vi "GetNI_SynthFocus_Bulk.vi"(0 "Digitizer Settings":T4={"Digitizer delay (us) "=0.0, "rf points per line"=2048, "lines per plane"=128, "Samp Rate (Hz)"=100000000.0, "Additional dig delay (us)"=0.0, "Voltage Scale"=0.4, "Pre-Looks"=0, "Offset delay (us)"=0.0, "bits A/D"=8, "Avg Num"=1, "DigTimeOut"=5.0, "Rel Dig Delay"=0.0, "Dig Ch"=0, "LeCroyCluster"={"LeCroy Channels"=[TRUE, FALSE, FALSE, FALSE], "LC read pt offset"=0.0, "Sweep Avg"=FALSE}, "Main Digitizer"=enum."NI Digitizer", "Dig Config"=enum."Single channel", "Digitizer ID Cluster"={"Acqiris/Alazar/SP ID"=[], "NI Instr Handles"=[], "LeCroy VISA"="", "GaGe Handle"={"Handle"=0, "Sample size"=0, "Resolution"=0, "Offset"=0, "Channels"=0, "Boards"=0}, "ATS Ref"="ATS9350", "Acqiris Address"=["PCI::INSTR0"], "ADQRef"=refnum, "adq_cu_ptr"=refnum}, "Trigger Settings"={"Trig Source"=1, "Trig Coupling"=0, "Trig Slope"=0, "Level (mV)"=1500.0}, "Bulk Acq"=FALSE, "Bulk Start Indexes"=[], "Data Ref RF"=refnum, "NI ID/Channel"=[], "Total Dig CH"=1, "Xtra Ann Trig delay (us)"=10.0, "Fix Z Delay?"=FALSE, "One Way Transmission?"=FALSE, "Data Ref Log"=refnum} {"Trigger Settings"."Trig Slope" items=["Positive", "Negative"]; "Trigger Settings"."Level (mV)" format="%.2f"; "Trigger Settings"."Trig Coupling" items=["DC 1 MOhm", "AC 1 MOhm", "DC 50 Ohm", "AC 50 Ohm"]; "Trigger Settings"."Trig Source" items=["Chan 1", "External"]; "Rel Dig Delay" format="%.2f"; "DigTimeOut" format="%.2f"; "Avg Num" min=1; "Offset delay (us)" format="%.2f"; "Additional dig delay (us)" format="%.2f"; "Digitizer delay (us)" format="%.2f"}, 5 "Ann Array Params":T1={"Synth Foc?"=FALSE, "Focal Zones"=41, "Switch T/R"=0, "Trans Geometry (mm)"={"Transducer"=0, "Geo Focus"=12.0, "a (radius)"=3.0, "# of rings"=5, "kerf space "=0.1, "Center Freq"=12.0}, "Sub Ap Excite?"=FALSE, "Full Array Scan?"=FALSE, "Xmt/Rcv"={"XMIT"=[TRUE, TRUE, TRUE, TRUE, TRUE], "RCV"=[TRUE, TRUE, TRUE, TRUE, TRUE]}, "PulseSpacing (us)"=0.0, "Xmit Ring"=0, "XMIT CHS"=0, "RCV CHS"=0, "GPU?"=FALSE, "Save TIFF?"=FALSE, "downfactor"=1, "RCV 1CH"=0} {"RCV 1CH" items=["All", "1", "2", "3", "4", "5"]; "Trans Geometry (mm)"."Transducer" items=["6D 12R 40 MHz"=0, "10D 31R 20 MHz"=1, "10D 23R 20 MHz"=2, "6D 23R 40 MHz"=3, "4.5D 10.7R 40 MHz"=4, "9D 23.5R 20 MHz"=5, "9D 25.8R 20MHz"=6, "Enter"=99]; "Switch T/R" min=1 max=5 step=1}, 7 "errorin":errorcluster, 8 "File Array":string[](array[string]), 10 "lines per plane":i32) -> (17 "Raw VGain (scale)":dbl, 18 "Gain Array":T8(array[cluster]), 21 "VGain (dB)":dbl, 27 "error out":errorcluster)   [LabVIEW 2022 SP3]
uses:
  -DigitizerRoutines/DigitizerSettings.ctl
  -DigitizerRoutines/Digitizer.ctl
  -DigitizerRoutines/DigConfig.ctl
  -DigitizerRoutines/DigitizerID.ctl
  C:/Windows/System32/ADQAPI_dotNet_helper.dll
  Annular Array/-AnnularRoutines/AnnularArray.ctl
  Annular Array/-AnnularRoutines/TransGeometry.ctl
  Annular Array/-AnnularRoutines/ArrayGeometry.ctl
  <instrlib>/niScope/Acquire/Fetch/niScope Multi Fetch Binary 8.vi
  -ScanSystem/DataHandling/ReverseDataI8.vi
  Annular Array/-SynthApperture/ProcImageHD_I8.vi
panel:
  out "read time":u32
  out "synth foc time":u32
  out "Numeric":i32
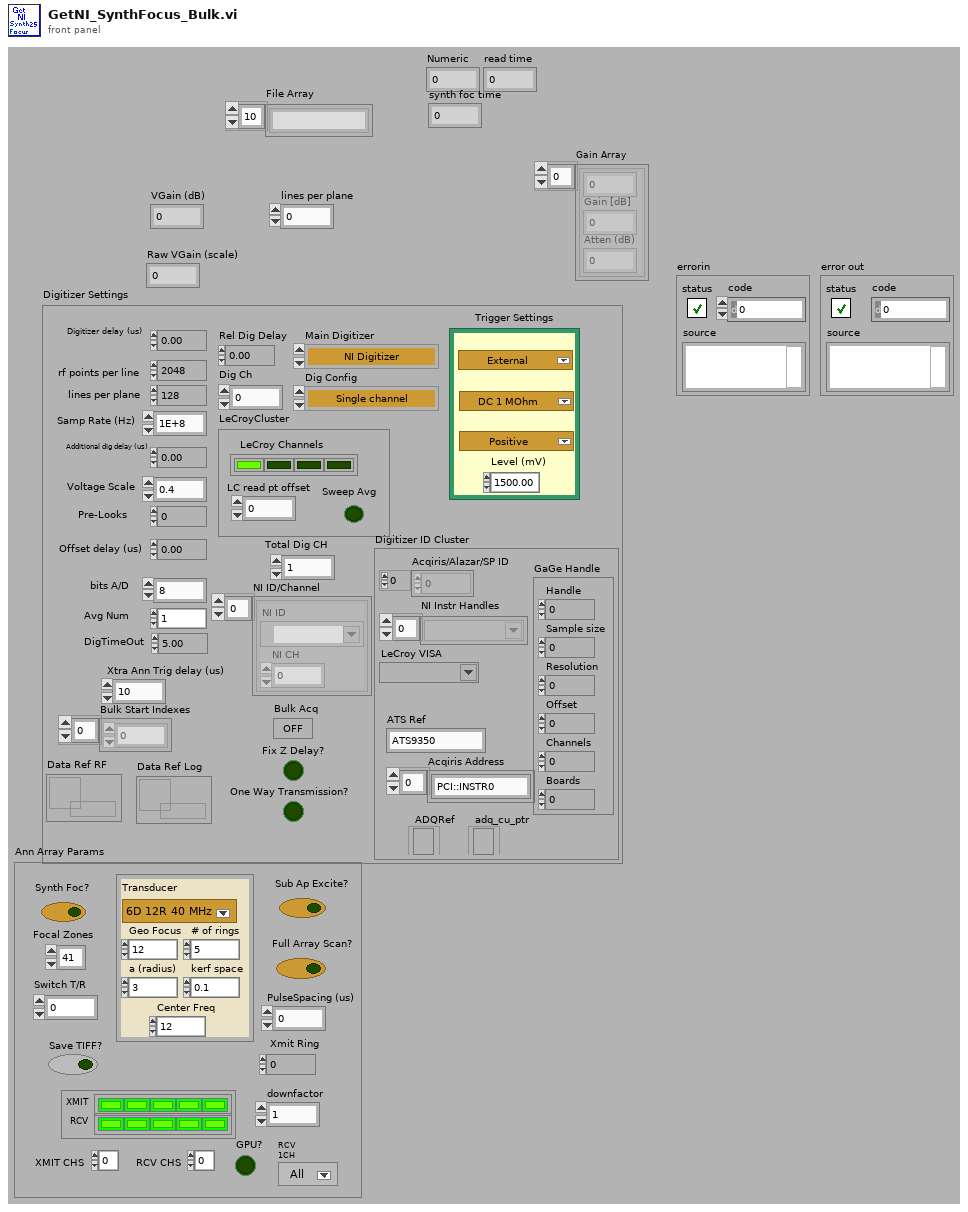
[diagram p1: front panel]
types:
  T1 = typedef "AnnularArray.ctl" = cluster{"Synth Foc?":bool, "Focal Zones":i16, "Switch T/R":i16, "Trans Geometry (mm)":T2, "Sub Ap Excite?":bool, "Full Array Scan?":bool, "Xmt/Rcv":cluster{"XMIT":bool[], "RCV":bool[]}, "PulseSpacing (us)":sgl, "Xmit Ring":i32, "XMIT CHS":u8, "RCV CHS":u8, "GPU?":bool, "Save TIFF?":bool, "downfactor":i32, "RCV 1CH":u16}
  T2 = typedef "TransGeometry.ctl" = cluster{"Transducer":T3, "Geo Focus":dbl, "a (radius)":dbl, "# of rings":i32, "kerf space ":dbl, "Center Freq":dbl}
  T3 = typedef "ArrayGeometry.ctl" = u16
  T4 = typedef "DigitizerSettings.ctl" = cluster{"Digitizer delay (us) ":dbl, "rf points per line":i32, "lines per plane":i32, "Samp Rate (Hz)":dbl, "Additional dig delay (us)":dbl, "Voltage Scale":dbl, "Pre-Looks":i32, "Offset delay (us)":dbl, "bits A/D":i8, "Avg Num":i32, "DigTimeOut":sgl, "Rel Dig Delay":sgl, "Dig Ch":i32, "LeCroyCluster":cluster{"LeCroy Channels":bool[], "LC read pt offset":dbl, "Sweep Avg":bool}, "Main Digitizer":T5, "Dig Config":T6, "Digitizer ID Cluster":T7, "Trigger Settings":cluster{"Trig Source":u16, "Trig Coupling":u16, "Trig Slope":u16, "Level (mV)":dbl}, "Bulk Acq":bool, "Bulk Start Indexes":i32[], "Data Ref RF":refnum<data-value>, "NI ID/Channel":cluster{"NI ID":refnum<k15>, "NI CH":i32}[], "Total Dig CH":i32, "Xtra Ann Trig delay (us)":dbl, "Fix Z Delay?":bool, "One Way Transmission?":bool, "Data Ref Log":refnum<data-value>}
  T5 = typedef "Digitizer.ctl" = enum16{"Acqiris Digitizer", "NI Digitizer", "LeCroy", "GaGe", "AlazarTech", "No Digitizer", "Teledyne"}
  T6 = typedef "DigConfig.ctl" = enum16{"Single channel", "2 Chans w/ 2 Acqiris", "2 Chans w/ 1 Acqiris", "5-CH Pulser New", "5-CH pulser w/ ann array", "5-pass style ann array", "Empty"}
  T7 = typedef "DigitizerID.ctl" = cluster{"Acqiris/Alazar/SP ID":u32[], "NI Instr Handles":refnum<k15>[], "LeCroy VISA":refnum<visa-resource-name>, "GaGe Handle":cluster{"Handle":u32, "Sample size":u32, "Resolution":i32, "Offset":i32, "Channels":u32, "Boards":u32}, "ATS Ref":string, "Acqiris Address":string[], "ADQRef":refnum<k24>, "adq_cu_ptr":refnum<k24>}
  T8 = cluster{sgl, "Gain [dB]  ":sgl, "Atten (dB)":sgl}[]
  T9 = cluster{"gain":dbl, "wfm":i8[][], "max queue size (-1, unlimited)":i32}
  T10 = cluster{"actualSamples":i32, "absoluteInitialX":dbl, "relativeInitialX":dbl, "xIncrement":dbl, "offset":dbl, "gain":dbl, "reserved1":dbl, "reserved2":dbl}[]
  T11 = cluster{"actualSamples":i32, "absoluteInitialX":dbl, "relativeInitialX":dbl, "xIncrement":dbl, "offset":dbl, "gain":dbl, "reserved1":dbl, "reserved2":dbl}
  T12 = cluster{sgl, "Gain [dB]  ":sgl, "Atten (dB)":sgl}
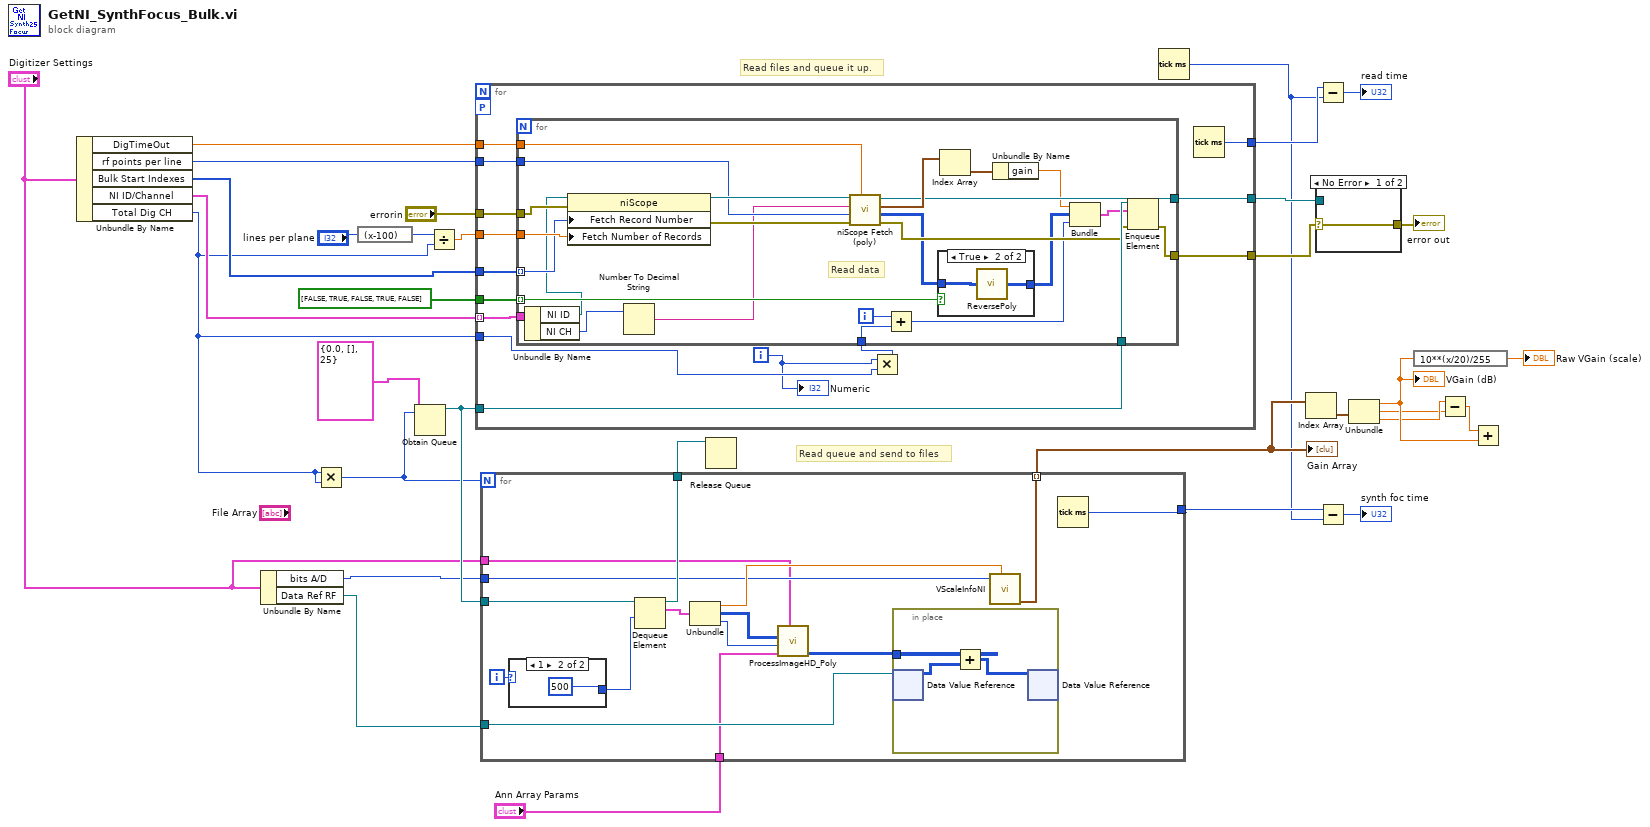
[diagram p0: block diagram]
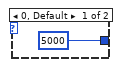
[diagram p2: hidden frame]
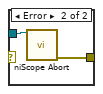
[diagram p3: hidden frame]
diagram:
  # "Read files and queue it up."
  # "Read queue and send to files"
  n1 = Unbundle By Name("Digitizer Settings") -> ("DigTimeOut"=w10:sgl, "rf points per line"=w12:i32, "Bulk Start Indexes"=w8:i32[], "NI ID/Channel"=w6:cluster{"NI ID":refnum<k15>, "NI CH":i32}[], "Total Dig CH"=w3:i32)
  n2 = Unbundle By Name("Digitizer Settings") -> ("bits A/D"=w11:i8, "Data Ref RF"=w7:refnum<data-value>)
  n3 = Multiply(x=w3, y=w3) -> (x*y=w2:i32)
  n4 = expression code="(x-100)"("lines per plane") -> (w5:i32)
  n5 = Obtain Queue(max queue size (-1, unlimited)=w2, element data type=T9 {"gain"=0.0, "wfm"=[], "max queue size (-1, unlimited)"=25}) -> (queue out=w22:refnum<queue>)  [unwired: 3 in, 2 out]
  n6 = Divide(x=w5, y=w3) -> (x/y=w4:dbl)
  n7 = for {
    tunnel: w10 -> [w47]
    tunnel: w12 -> [w44]
    tunnel: "errorin" -> [w46]
    tunnel: w4 -> [w37]
    tunnel: [w45] -> w31
    tunnel: w22 -> [w43]
    tunnel: [w42] -> w21
    tunnel: [w41] -> w20
    tunnel: w8 -> [w40]
    tunnel: bool[] [FALSE, TRUE, FALSE, TRUE, FALSE] -> [w39]
    workers-P: _ -> [_]
    tunnel: w6 -> [w38] mode=indexing
    tunnel: w3 -> [w36]
    i -> [w34]
    n8 = Multiply(x=w34, y=w36) -> (x*y=w35:i32)
    n9 = for {
      tunnel: w47 -> [w72]
      tunnel: w46 -> [w71]
      tunnel: w37 -> [w67]
      tunnel: [w66] -> w45
      tunnel: w44 -> [w64]
      tunnel: w43 -> [w63]
      tunnel: [w59] -> w42
      tunnel: w40 -> [w61] mode=indexing
      tunnel: w35 -> [w56]
      tunnel: w39 -> [w54] mode=indexing
      tunnel: w38 -> [w51]
      i -> [w55]
      # "Read data"
      n10 = Unbundle By Name(w51) -> ("NI ID"=w50:refnum<k15>, "NI CH"=w49:i32)
      n11 = property class="niScope"(reference=w50, error in=w71, "Fetch Record Number"=w61, "Fetch Number of Records"=w67) -> (reference out=w65:refnum<k15>, error out=w70:errorcluster)
      n12 = Number To Decimal String(number=w49) -> (decimal integer string=w48:string)  [unwired: 1 out]
      n13 = call-poly <instrlib>:"niScope Fetch (poly).vi"("timeout"=w72, "error in"=w70, "numSamples"=w64, "channels"=w48, "instrument handle"=w65) -> ("error out"=w60:errorcluster, "wfm"=w58:i8[][], "wfm info"=w69:T10, "instrument handle out"=w66:refnum<k15>)  [unwired: 3 out]
      n14 = Add(x=w55, y=w56) -> (x+y=w53:i32)
      n15 = case shown="True" w54 {
        tunnel: w58 -> [w73 w75]
        tunnel: [w73 w74] -> w57
        frame False {
        }
        frame True {
          n16 = call-poly "ReversePoly.vi"("Array in"=w75) -> ("Array out"=w74:i8[][])
        }
      }
      n17 = Index Array(array=w69) -> (element=w68:T11)  [unwired: 1 in]
      n18 = Unbundle By Name(w68) -> ("gain"=w62:dbl)
      n19 = Bundle("gain"=w62, "Array out"=w57, w53) -> (w52:cluster{"gain":dbl, "Array out":i8[][], i32})  [unwired: 1 in]
      n20 = Enqueue Element(queue=w63, element=w52, error in (no error)=w60) -> (error out=w59:errorcluster)  [unwired: 1 in, 2 out]
    }
    n21 = Tick Count (ms)() -> (millisecond timer value=w41:u32)
    "Numeric" <- w34
  }
  n22 = for {
    N: w2 -> [_]
    tunnel: [w90] -> w23 mode=indexing
    tunnel: w22 -> [w89]
    tunnel: [w85] -> w15
    tunnel: [w84] -> w19
    tunnel: w7 -> [w83]
    tunnel: w11 -> [w78]
    tunnel: "Digitizer Settings" -> [w77]
    tunnel: "Ann Array Params" -> [w76]
    i -> [w80]
    n23 = case shown="1" w80 {
      tunnel: [5000 500] -> w79
      frame 0, Default {
      }
      frame 1 {
      }
    }
    n24 = Dequeue Element(queue=w89, timeout in ms (-1)=w79) -> (queue out=w85:refnum<queue>, element=w88:T9)  [unwired: 1 in, 2 out]
    n25 = Unbundle(w88) -> ("gain"=w87:dbl, "wfm"=w86:i8[][], "max queue size (-1, unlimited)"=w81:i32)
    n26 = call-poly "ProcessImageHD_Poly.vi"("Digitizer Settings"=w77, "Ann Array Params"=w76, "T/R Ring"=w81, "Scan Data In"=w86) -> ("Synth App Out"=w82:i16[][])  [unwired: 4 in, 1 out]
    n27 = in-place {
      in-place-border: w82 -> [w93]
      n28 = in-place-dvr #1(w83) -> (w95:i16[][])  [unwired: 1 out]
      n29 = Add(x=w93, y=w95) -> (x+y=w94:i16[][])
      n30 = in-place-dvr #1(w94) -> ()  [unwired: 2 out]
    }
    n31 = call "VScaleInfoNI.vi"("A/D bits"=w78, "gain"=w87) -> ("Voltage Scale"=w90:T12)  [unwired: 5 in, 3 out]
    n32 = Tick Count (ms)() -> (millisecond timer value=w84:u32)
  }
  "Gain Array" <- w23
  n33 = Release Queue(queue=w15) -> ()  [unwired: 2 in, 3 out]
  n34 = Tick Count (ms)() -> (millisecond timer value=w18:u32)
  n35 = Index Array(array=w23) -> (element=w30:T12)  [unwired: 1 in]
  n36 = case shown="No Error" w21 {
    selector: w21 -> [w96 _]
    tunnel: w31 -> [_ w98]
    tunnel: [w96 w97] -> w32
    frame No Error {
    }
    frame Error {
      n37 = call <instrlib>:"niScope Abort.vi"("instrument handle"=w98) -> ("error out"=w97:errorcluster)  [unwired: 1 in, 13 out]
    }
  }
  "error out" <- w32
  n38 = Subtract(x=w20, y=w18) -> (x-y=→"read time":u32)
  n39 = Subtract(x=w19, y=w18) -> (x-y=→"synth foc time":u32)
  n40 = Unbundle(w30) -> (w29:sgl, "Gain [dB]"=w27:sgl, "Atten (dB)"=w28:sgl)
  "VGain (dB)" <- w29
  n41 = expression code="10**(x/20)/255"(w29) -> (→"Raw VGain (scale)":sgl)
  n42 = Subtract(x=w28, y=w27) -> (x-y=w26:sgl)
  n43 = Add(x=w26, y=w29) -> ()  [unwired: 1 out]
